vi "Add Multiple Symbol Notifications.vi"(7 "Aliases":string[](array[string]), 8 "error in (no error)":errorcluster, 9 "Cycle Time (ms)":i32, 10 "Symbol Names":string[](array[string]), 11 "TwinCAT ADS in":refnum<class "TwinCAT ADS.lvclass">) -> (0 "error out":errorcluster, 3 "TwinCAT ADS out":refnum<class "TwinCAT ADS.lvclass">)   [LabVIEW 2018, in "TwinCAT ADS.lvclass"]
uses:
  TwinCAT ADS.lvclass
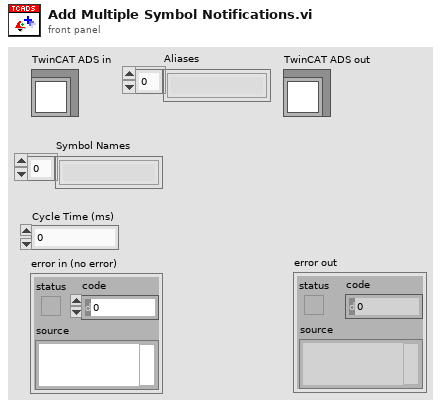
[diagram p1: front panel]
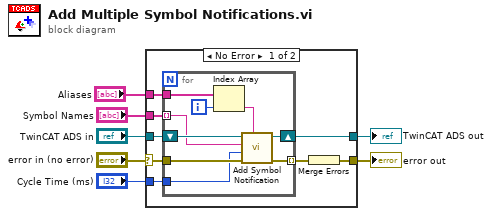
[diagram p0: block diagram]
diagram:
  n1 = case shown="No Error" "error in (no error)" {
    selector: "error in (no error)" -> [w8 w26]
    tunnel: [w10 w26] -> w6
    tunnel: [w11 w25] -> w4
    tunnel: "TwinCAT ADS in" -> [w15 w25]
    tunnel: "Cycle Time (ms)" -> [w13 _]
    tunnel: "Symbol Names" -> [w14 _]
    tunnel: "Aliases" -> [w9 _]
    frame No Error {
      n2 = for {
        shift-right: [w23] -> w11
        shift-left: w15 -> [w24]
        tunnel: [w22] -> w12 mode=indexing
        tunnel: w14 -> [w21] mode=indexing
        tunnel: w13 -> [w19]
        tunnel: w9 -> [w18]
        tunnel: w8 -> [w20]
        i -> [w17]
        n3 = Index Array(array=w18, index=w17) -> (element=w16:string)
        n4 = call "Add Symbol Notification.vi"("Alias"=w16, "error in (no error)"=w20, "Cycle Time (ms)"=w19, "Symbol Name"=w21, "TwinCAT ADS in"=w24) -> ("error out"=w22:errorcluster, "TwinCAT ADS out"=w23:refnum<class "TwinCAT ADS.lvclass">)  [unwired: 5 in]
      }
      n5 = Merge Errors(w12) -> (w10:errorcluster)
    }
    frame Error {
    }
  }
  "error out" <- w6
  "TwinCAT ADS out" <- w4
